vi "AddStepToTree.vi"(11 "Step":T1) -> (0 "error out":errorcluster)   [LabVIEW 2015]
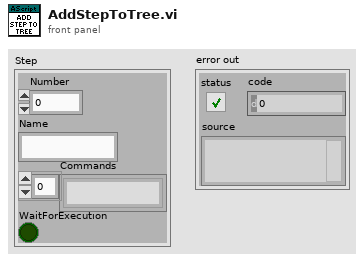
[diagram p1: front panel]
types:
  T1 = cluster{"Number":i32, "Name":string, "Commands":string[], "WaitForExecution":bool}
  T2 = cluster{"Return Variable Names":refnum<vi>, "ArgumentsBox":refnum<vi>, "Routine":refnum<vi>, "AddCmd":refnum<vi>, "ClearSteps":refnum<vi>, "AddStep":refnum<vi>, "DeleteAuto":refnum<vi>, "DeleteCommand":refnum<vi>, "DeleteStep":refnum<vi>, "TemplateOpen":refnum<vi>, "SaveStep":refnum<vi>, "LoadAuto":refnum<vi>, "SaveAuto":refnum<vi>, "LoadStep":refnum<vi>, "AutoFiles":refnum<vi>, "DeleteLog":refnum<vi>, "GetLogFile":refnum<vi>, "Auto Script on Robot":refnum<vi>, "DLfromRIO":refnum<vi>, "Autoscript Layout":refnum<vi>, "Auto Script Name":refnum<vi>, "ULtoRIO":refnum<vi>}
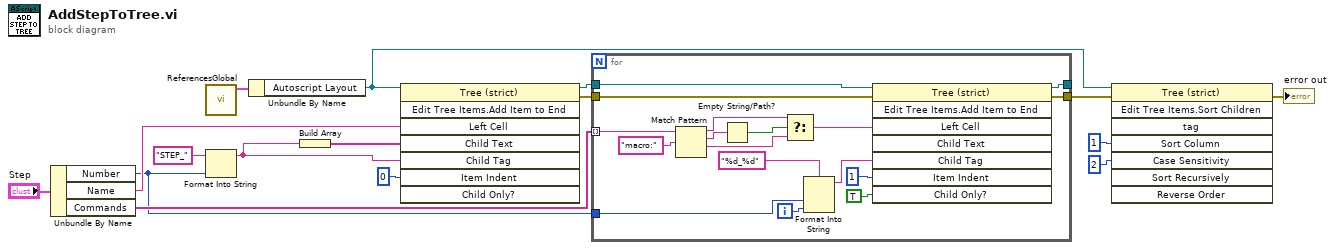
[diagram p0: block diagram]
diagram:
  n1 = Unbundle By Name("Step") -> ("Number"=w8:i32, "Name"=w13:string, "Commands"=w12:string[])
  n2 = call "ReferencesGlobal.vi"() -> ("AscriptRefsOut"=w1:T2)  [unwired: 11 in]
  n3 = Format Into String(initial string="STEP_", w8) -> (resulting string=w10:string)  [unwired: 2 in, 1 out]
  n4 = Unbundle By Name(w1) -> ("Autoscript Layout"=w3:refnum<vi>)
  n5 = Build Array(w10) -> (w14:string[])
  n6 = invoke class="Tree (strict)" method="Edit Tree Items.Add Item to End"(reference=w3, "Left Cell"=w13, "Child Text"=w14, "Child Tag"=w10, "Item Indent"=0 ("New Item Indentation")) -> (reference out=w11:refnum<vi>, error out=w6:errorcluster)  [unwired: 3 in, 6 out]
  n7 = for {
    tunnel: w11 -> [w33]
    tunnel: w12 -> [w26] mode=indexing
    tunnel: w8 -> [w30]
    tunnel: [w19] -> _
    tunnel: w6 -> [w18]
    tunnel: [w17] -> w2
    i -> [w29]
    n8 = Match Pattern(string=w26, regular expression="macro:") -> (before substring=w22:string, match substring=w24:string, after substring=w21:string)  [unwired: 1 in, 1 out]
    n9 = Empty String/Path?(string/path=w24) -> (empty?=w23:bool)
    n10 = Select(t=w22, s=w23, f=w21) -> (s? t:f=w20:string)
    n11 = Format Into String(format string="%d_%d", w30, w29) -> (resulting string=w28:string)  [unwired: 2 in, 1 out]
    n12 = invoke class="Tree (strict)" method="Edit Tree Items.Add Item to End"(reference=w33, error in=w18, "Left Cell"=w20, "Child Tag"=w28, "Item Indent"=1 ("New Item Indentation"), "Child Only?"=TRUE) -> (reference out=w19:refnum<vi>, error out=w17:errorcluster)  [unwired: 2 in, 6 out]
  }
  n13 = invoke class="Tree (strict)" method="Edit Tree Items.Sort Children"(reference=w3, error in=w2, "Sort Column"=1, "Case Sensitivity"=2) -> (error out=→"error out":errorcluster)  [unwired: 4 in, 7 out]
